vi "Read Limit Test Result.vi"(8 "error in (no error)":errorcluster, 10 "Timeout (10000 ms)":u32=10000, 11 "VISA resource name":refnum<visa-resource-name>) -> (0 "error out":errorcluster, 1 "Upper Limit Test Fail?":bool, 2 "Lower Limit Test Fail?":bool, 3 "VISA resource name out":refnum<visa-resource-name>)   [LabVIEW 2021, in "Agilent 532XX Series.lvlib"]
doc: "Performs a single, new measurement and outputs limit test results."
uses:
  <instrlib>/Agilent 532XX Series/Agilent 532XX Series.lvlib
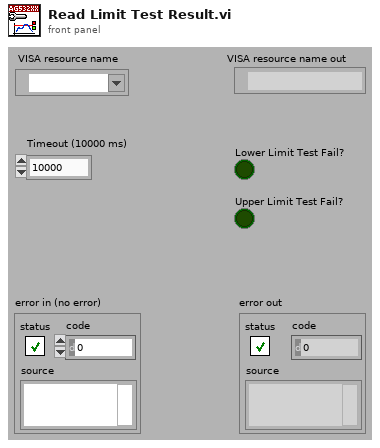
[diagram p1: front panel]
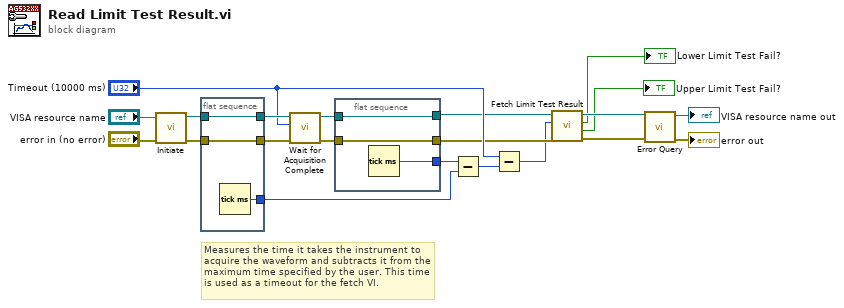
[diagram p0: block diagram]
diagram:
  # "Measures the time it takes the instrument to acquire the waveform and subtracts it from the maximum time specified by the user. This time is used as a timeout for the fetch VI."
  n1 = call <instrlib>:"Initiate.vi"("error in (no error)"="error in (no error)", "VISA resource name"="VISA resource name") -> ("error out"=w15:errorcluster, "VISA resource name out"=w16:refnum<visa-resource-name>)  [unwired: 8 out]
  n2 = flat-sequence {
    tunnel: [w24] -> w12
    tunnel: w16 -> [w24]
    tunnel: [w23] -> w13
    tunnel: w15 -> [w23]
    tunnel: [w22] -> w14
    frame #0 {
      n3 = Tick Count (ms)() -> (millisecond timer value=w22:u32)
    }
  }
  n4 = call <instrlib>:"Wait for Acquisition Complete.vi"("error in (no error)"=w13, "Maximum Time (10000 ms)"="Timeout (10000 ms)", "VISA resource name"=w12) -> ("error out"=w9:errorcluster, "VISA resource name out"=w10:refnum<visa-resource-name>)  [unwired: 1 in, 6 out]
  n5 = flat-sequence {
    tunnel: [w27] -> w5
    tunnel: w10 -> [w27]
    tunnel: [w26] -> w4
    tunnel: w9 -> [w26]
    tunnel: [w25] -> w8
    frame #0 {
      n6 = Tick Count (ms)() -> (millisecond timer value=w25:u32)
    }
  }
  n7 = Subtract(x=w8, y=w14) -> (x-y=w17:u32)
  n8 = Subtract(x="Timeout (10000 ms)", y=w17) -> (x-y=w3:u32)
  n9 = call <instrlib>:"Fetch Limit Test Result.vi"("error in (no error)"=w4, "Timeout (10000 ms)"=w3, "VISA resource name"=w5) -> ("error out"=w7:errorcluster, "Upper Limit Test Fail ?"=→"Upper Limit Test Fail?":bool, "Lower Limit Test Fail ?"=→"Lower Limit Test Fail?":bool, "VISA resource name out"=w6:refnum<visa-resource-name>)  [unwired: 5 out]
  n10 = call <instrlib>:"Error Query.vi"("error in (no error)"=w7, "VISA resource name"=w6) -> ("error out"=→"error out":errorcluster, "VISA resource name out"=→"VISA resource name out":refnum<visa-resource-name>)  [unwired: 8 out]
